vi "Anthony-Sandoval-Lab5-part-2.vi"() -> ()   [LabVIEW 2010]
uses:
  <vilib>/Utility/file.llb/Write To Spreadsheet File (I64).vi
panel:
  in  "File path ending":string
  out "date/time string":string
  in  "time format string (%c)":string
  in  "Save":bool
  out "Old Graph":u16[](graph)
  out "Actual sample Rate":i32
  out "New Graph":u16[](graph)
  out "ErrMsg":string
  out "ErrCode":i32
  in  "LowChan":i32
  in  "HighChan":i32
  in  "number of samples to be collected":i32=5000
  in  "Sampling Rate in samples/sec.":i32=8000
  in  "Range":i32(ring)=2 items=["Not Programmable"=0, "+- 20 V"=27, "+- 10 V"=1, "+- 5 V"=2, "+- 4 V"=28, "+- 2.5 V"=3, "+- 2 V"=29, "+- 1.67 V"=4, "+- 1.25 V"=5, "+- 1 V"=6, "+- .625 V"=7, "+- .5 V"=8, "+- .25 V"=30, "+- .2 V"=31, "+- .1 V"=9, "+- .05 V"=10, "+- .01 V"=11, "+- .005 V"=12, "0 - 10 V"=13, "0 - 5 V"=14, "0 - 4 V"=36, "0 - 2.5 V"=15, "0 - 2 V"=16, "0 - 1.67 V"=17, "0 - 1.25 V"=18, "0 - 1 V"=19, "0 - .5 V"=32, "0 - .25 V"=33, "0 - .2 V"=34, "0 - .1 V"=20, "0 - .02 V"=35, "0 - .01 V"=21, "4 - 20 mA"=22, "2 - 10 mA"=23, "1 - 5 mA"=24, ".5 - 2.5 mA"=25, "0 - 20 mA"=26]
  in  "Options":i32
  in  "InterChannel Delay":sgl=-1.0 format="%.2f"
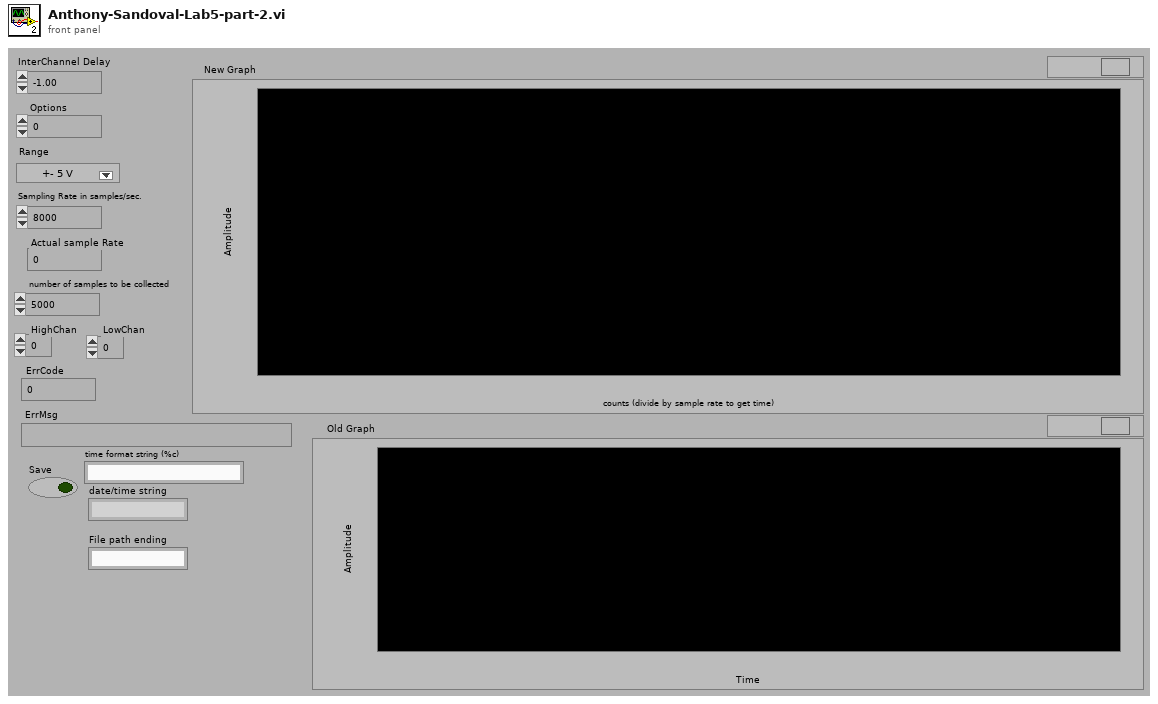
[diagram p1: front panel]
types:
  T1 = typedef "imagedata.ctl" = cluster{"image type":i32, "image depth":i32, "image":u8[], "mask":u8[], "colors":u32[], "Rectangle":cluster{"left":i16, "top":i16, "right":i16, "bottom":i16}}
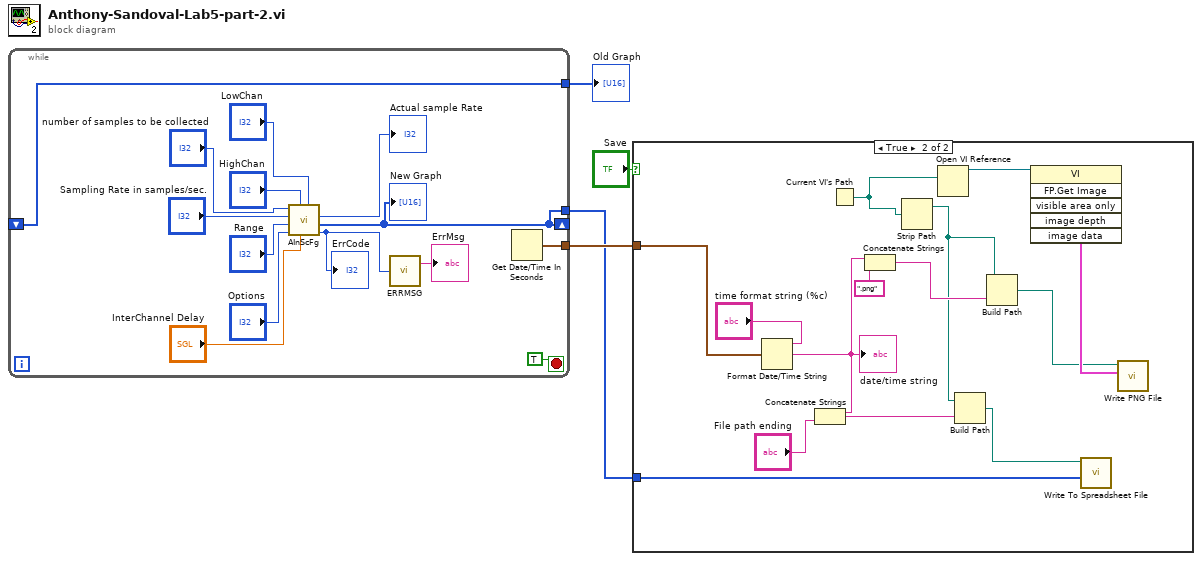
[diagram p0: block diagram]
diagram:
  n1 = while {
    shift-right: [w6] -> _
    shift-left: _ -> [w5]
    tunnel: [w7] -> w3
    tunnel: [w6] -> w1
    tunnel: [w5] -> w2
    stop <- TRUE stop-if-true
    n2 = call <menus>:"AInScFg.VI"("LowChan"="LowChan", "InterChannel Delay"="InterChannel Delay", "HighChan"="HighChan", "Options"="Options", "Range"="Range", "Rate"="Sampling Rate in samples/sec.", "Count"="number of samples to be collected") -> ("ErrCode"=w11:i32, "ADData"=w6:u16[], "Rate"=→"Actual sample Rate":i32)  [unwired: 1 in]
    "ErrCode" <- w11
    "New Graph" <- w6
    n3 = call <menus>:"ERRMSG.VI"("ErrCode"=w11) -> ("ErrMsg"=→"ErrMsg":string)  [unwired: 1 out]
    n4 = Get Date/Time In Seconds() -> (seconds since 1Jan1904=w7:timestamp)
  }
  "Old Graph" <- w2
  n5 = case shown="True" "Save" {
    tunnel: w3 -> [_ w32]
    tunnel: w1 -> [_ w19]
    frame False {
    }
    frame True {
      n6 = Format Date/Time String(time format string (%c)="time format string (%c)", seconds (now)=w32) -> (date/time string=w28:string)  [unwired: 1 in]
      "date/time string" <- w28
      n7 = Concatenate Strings(w28, "File path ending") -> (w29:string)
      n8 = Current VI's Path() -> (path=w22:path)
      n9 = Concatenate Strings(w28, ".png" ("File extension")) -> (w24:string)
      n10 = Strip Path(path=w22) -> (stripped path=w21:path)  [unwired: 1 out]
      n11 = Open VI Reference(vi path=w22) -> (vi reference=w26:refnum<vi>)  [unwired: 5 in, 1 out]
      n12 = Build Path(base path=w21, name or relative path=w29) -> (appended path=w20:path)
      n13 = Build Path(base path=w21, name or relative path=w24) -> (appended path=w23:path)
      n14 = invoke class="VI" method="FP.Get Image"(reference=w26) -> ("image data"=w25:T1)  [unwired: 5 in, 5 out]
      n15 = call-poly <vilib>:"Write To Spreadsheet File.vi"("1D data"=w19, "file path (dialog if empty)"=w20) -> ()  [unwired: 6 in, 1 out]
      n16 = call <vilib>:"Write PNG File.vi"("image data"=w25, "path to PNG file"=w23) -> ()  [unwired: 8 in, 2 out]
    }
  }
